vi "Cluster - Write Age.vi"(8 "error in (no error)":errorcluster, 11 "ClusterWithClass":T2) -> (0 "error out":errorcluster, 3 "ClusterWithClass Out":T2)   [LabVIEW 2012]
uses:
  ClassDefinitions/SimpleClassWithProperties/myClass.lvclass
panel:
  in  "Cluster":T1
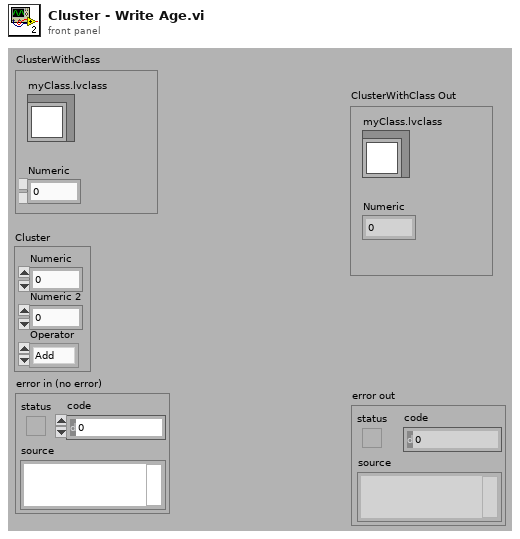
[diagram p1: front panel]
types:
  T1 = cluster{"Numeric":dbl, "Numeric 2":dbl, "Operator":enum16{"Add", "Divide", "Multiple", "Subtract"}}
  T2 = cluster{"myClass.lvclass":refnum<class "myClass.lvclass">, "Numeric":dbl}
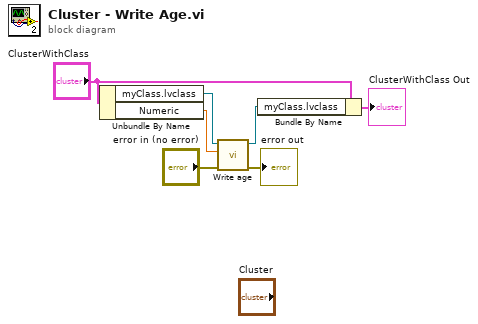
[diagram p0: block diagram]
diagram:
  n1 = Unbundle By Name("ClusterWithClass") -> ("myClass.lvclass"=w7:refnum<class "myClass.lvclass">, "Numeric"=w6:dbl)
  n2 = call-dynamic "Write age.vi"("error in (no error)"="error in (no error)", "age"=w6, "myClass in"=w7) -> ("error out"=→"error out":errorcluster, "myClass out"=w3:refnum<class "myClass.lvclass">)  [unwired: 7 in]
  n3 = Bundle By Name(cluster="ClusterWithClass", "myClass.lvclass"=w3) -> (→"ClusterWithClass Out":T2)
